vi "PATCH.vi"(8 "error in":errorcluster, 10 "httpRequest":refnum<class "httpRequest.lvclass">, 11 "http-client in":refnum<class "httpClient.lvclass">) -> (0 "error out":errorcluster, 2 "httpResponse":refnum<class "httpResponse.lvclass">, 3 "http-client out":refnum<class "httpClient.lvclass">)   [LabVIEW 2020, in "httpClient.lvlib" / "httpClient.lvclass"]
uses:
  httpClient.lvclass
  httpRequest/httpRequest.lvclass
  httpResponse/httpResponse.lvclass
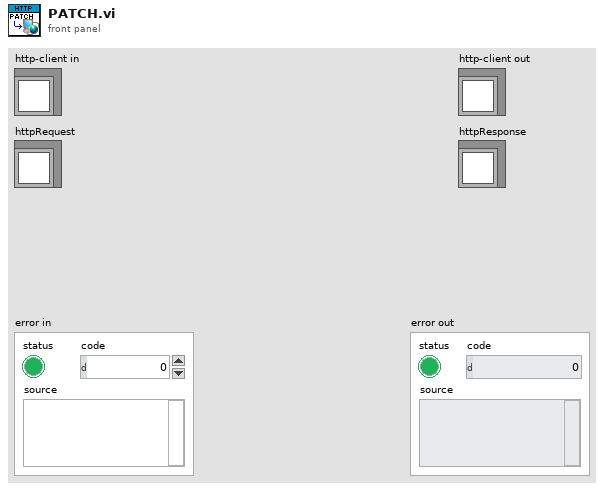
[diagram p1: front panel]
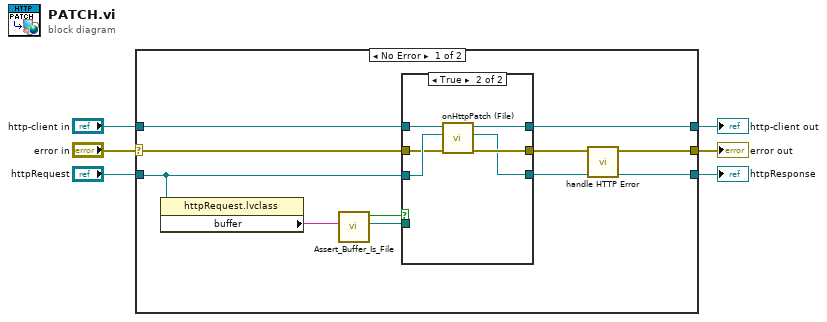
[diagram p0: block diagram]
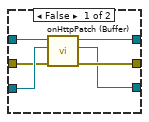
[diagram p2: hidden frame]
diagram:
  n1 = case shown="No Error" "error in" {
    selector: "error in" -> [w13 w31]
    tunnel: [w11 w31] -> w5
    tunnel: [w14 w30] -> w3
    tunnel: "http-client in" -> [w15 w30]
    tunnel: [w7 _] -> w2
    tunnel: "httpRequest" -> [w9 _]
    frame No Error {
      n2 = property class="httpRequest.lvclass"(reference=w9) -> ("buffer"=w10:string)  [unwired: 1 in, 2 out]
      n3 = call "Assert_Buffer_Is_File.vi"("buffer"=w10) -> ("File"=w16:path, "is File?"=w17:bool)  [unwired: 9 in]
      n4 = case shown="True" w17 {
        tunnel: w16 -> [_ _]
        tunnel: w15 -> [w18 w29]
        tunnel: [w23 w25] -> w14
        tunnel: [w21 w24] -> w8
        tunnel: w9 -> [w20 w28]
        tunnel: [w22 w26] -> w12
        tunnel: w13 -> [w19 w27]
        frame False {
          n5 = call-dynamic "onHttpPatch (Buffer).vi"("error in"=w19, "httpRequest"=w20, "http-client in"=w18) -> ("error out"=w22:errorcluster, "httpResponse"=w21:refnum<class "httpResponse.lvclass">, "http-client out"=w23:refnum<class "httpClient.lvclass">)  [unwired: 6 in]
        }
        frame True {
          n6 = call-dynamic "onHttpPatch (File).vi"("error in"=w27, "httpRequest"=w28, "http-client in"=w29) -> ("error out"=w26:errorcluster, "httpResponse"=w24:refnum<class "httpResponse.lvclass">, "http-client out"=w25:refnum<class "httpClient.lvclass">)  [unwired: 6 in]
        }
      }
      n7 = call "handle HTTP Error.vi"("httpResponse"=w8, "error in (no error)"=w12) -> ("httpResponse out"=w7:refnum<class "httpResponse.lvclass">, "error out"=w11:errorcluster)  [unwired: 8 in]
    }
    frame Error {
    }
  }
  "error out" <- w5
  "http-client out" <- w3
  "httpResponse" <- w2
